vi "Dashboard Main.vi"() -> ()   [LabVIEW 2016]
uses:
  Shared/PID Settings.ctl
  <vilib>/Utility/miscctls.llb/LVRowAndColumnTypeDef.ctl
  <vilib>/event_ctls.llb/eventvkey.ctl
  <vilib>/Rock Robotics/Network Tables/NT Read Numeric Array.vi
  <vilib>/Rock Robotics/WPI/Dashboard/WPI_DashboardLogging Global.vi
panel:
  in  "Camera Settings Right":T1={"Frame Rate"=30, "Compression"=30, "Size"=1, "DB Camera Config"=FALSE} {"Frame Rate" scale=1.0..30.0; "Compression" scale=100.0..-1.0; "Size" items=["640x480", "320x240", "160x120"]}
  in  "Camera Name Right":string(combo)="No Camera Selection"
  out "Camera Info":cluster{"Mbps LED":bool, "Mbps":dbl, "fps":dbl} {"fps" format="%#.1g"; "Mbps" format="%#.1g"}
  in  "Camera Settings":T1={"Frame Rate"=30, "Compression"=30, "Size"=1, "DB Camera Config"=FALSE} {"Frame Rate" scale=1.0..30.0; "Compression" scale=100.0..-1.0; "Size" items=["640x480", "320x240", "160x120"]}
  in  "TCP":refnum<k5>
  in  "Rec Mode":enum32{"Stop", "Record", "Playback"}(radio)
  out "Robot IP":string
  out "Image Message":string="Timeout in Camera Communications"
  in  "Dashboard Tab":T2(tab)
  in  "Select Auto":string(combo)="Select Autonomous ..."
  out "NT Connection":bool
  out "MotorChart R":cluster{"Numeric":dbl, "Numeric":dbl}(graph)
  out "MotorChart L":cluster{"Numeric":dbl, "Numeric":dbl}(graph)
  out "MotorSliders R":cluster{"MotorSlide1":dbl, "MotorSlide2":dbl} {"MotorSlide2" scale=-1.0..1.0 scale format="%#_2e"; "MotorSlide1" scale=-1.0..1.0 scale format="%#_2e"}
  out "MotorSliders L":cluster{"MotorSlide1":dbl, "MotorSlide2":dbl} {"MotorSlide2" scale=-1.0..1.0 scale format="%#_2e"; "MotorSlide1" scale=-1.0..1.0 scale format="%#_2e"}
  out "Gyro":dbl(knob) scale=0.0..360.0
  out "JS1 Z":dbl(slide) scale=-1.0..1.0 scale format="%#_2e"
  out "JS1 Graph":cluster{"X":dbl, "Y":dbl}[](graph)
  out "JS1 Buttons":T3
  out "JS2 Z":dbl(slide) scale=-1.0..1.0 scale format="%#_2e"
  out "JS2 Graph":cluster{"X":dbl, "Y":dbl}[](graph)
  out "JS2 Buttons":T3
  out "Mode":T4(ring)=enum."Auto Disabled"
  out "Camera Image Right":T5(plugin-control)
  in  "DB/String 9":string
  in  "DB/String 8":string
  in  "DB/String 7":string
  in  "DB/String 6":string
  in  "DB/String 5":string
  in  "DB/String 4":string
  in  "DB/String 3":string
  in  "DB/String 2":string
  in  "DB/String 1":string
  in  "DB/String 0":string
  in  "DB/Slider 0":dbl(slide) scale=0.0..5.0
  in  "DB/Slider 1":dbl(slide) scale=0.0..5.0
  in  "DB/Slider 2":dbl(slide) scale=0.0..5.0
  in  "DB/Slider 3":dbl(slide) scale=0.0..5.0
  out "DB/LED 3":bool
  out "DB/LED 2":bool
  out "DB/LED 1":bool
  out "DB/LED 0":bool
  in  "DB/Button 3":bool
  in  "DB/Button 2":bool
  in  "DB/Button 1":bool
  in  "DB/Button 0":bool caption="New Name"
  in  "Custom Tab Control":enum32{"Basic", "Robot Drive"}(tab)
  in  "Save Values":bool
  in  "Drive PID - High":T6
  in  "Left / Right":bool
  out "PID Graph":cluster{"Numeric":dbl, "Numeric":dbl}(graph)
  in  "Drive PID - Low":T6
  in  "Test Slider":dbl(slide) scale=0.0..100.0 scale format="%#_3g"
  in  "On/Off":bool caption="Solenoid"
  in  "Test Name":u16(ring) items=["Select the test to run..."]
  in  "Test Tree":string(tree)
  in  "Motor":cluster{"Value":dbl, "Enable":bool} {"Value" scale=-1.0..1.0 scale format="%#_3g"}
  out "Progress":T7 {"Test Progress" scale=0.0..100.0}
  in  "Rev/Fwd":cluster{"Forward":bool, "Reverse":bool}
  in  "Test Ring":u16(ring) items=["Monochrome", "Color"]
  out "Cmd Status":string
  in  "Execute Command":bool
  in  "Command Params":string[][](table)
  in  "Command Selection":i32(listbox)
  in  "CheckList":i32(listbox)
  out "Tree":string(tree)
  out "Camera Image":T5(plugin-control)
  out "Background":bool
  in  "Camera Name":string(combo)="No Camera Selection"
  # "HW"
  # "HW"
  # "Joysticks"
  # "Drive Motors"
  # "Front"
  # "Right"
  # "Left"
  # "Back"
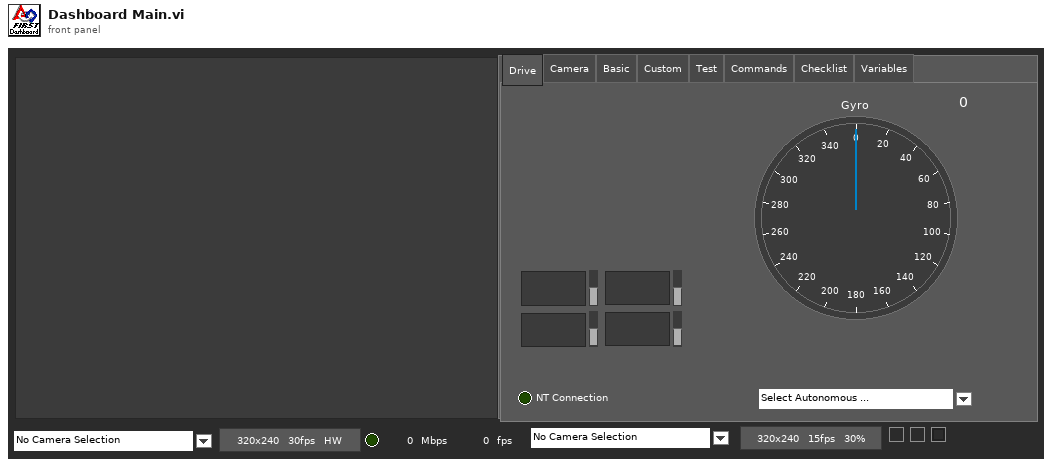
[diagram p1: front panel]
types:
  T1 = cluster{"Frame Rate":i32, "Compression":i32, "Size":u16, "DB Camera Config":bool}
  T2 = enum32{"Drive", "Camera", "Basic", "Custom", "Test", "Commands", "Checklist", "Variables"}
  T3 = cluster{bool, bool, bool, bool, bool, bool, bool, bool, bool, bool, bool, bool}
  T4 = enum8{"Tele-Op Disabled", "Tele-Op Enabled", "Auto Disabled", "Auto Enabled", "Test Disabled", "Test Enabled", "Disconnected", "No Code", "E-Stop"}
  T5 = typedef "IMAQ Image.ctl" = refnum<image>
  T6 = typedef "PID Settings.ctl" = cluster{"D":dbl, "F":dbl, "RR":dbl, "IZ":dbl, "P":dbl, "I":dbl}
  T7 = cluster{"Test Progress":u8, "Test Progress Text":string}
  T8 = typedef "Image Type" = u32
  T9 = cluster{"IDs":cluster{"RPC field ID":u16, "Unique ID":u16}, "String":string}
  T10 = enum32{"Drive", "Basic", "Custom", "Test", "Checklist", "Variables"}
  T11 = cluster{"Error Strings":string, "Disable Counts":cluster{u16, u16}, "Rail Faults":cluster{u16, u16, u16}, "Robot IP":string, "DB Mode":u8, "Event Info":cluster{"Name":string, "Type":u8, "Number":u16, "Replay":u8}}
  T12 = cluster{"Storage":cluster{"Disk Free":u64, "RAM Block":u32, "RAM free":u32}, "CPU Utilization":cluster{"CPU % ISR":sgl, "CPU % Time Crit":sgl, "CPU % Timed Str":sgl, "CPU % High":sgl, "CPU % Above":sgl, "CPU % Normal":sgl, "CPU % Low":sgl}, "CAN":cluster{"% Bus Utilization":sgl, "Bus Off Cnt":u32, "TX_FIFO Full Cnt":u32, "Receive Error Cnt":u8, "Transmit Error Cnt":u8}, "HID":cluster{"HID Outputs":u32, "Rumble Low":u16, "Rumble High":u16}[]}
  T13 = cluster{"Status bits":cluster{"Test Mode":bool, "Autonomous":bool, "Enabled":bool, "Code Start":bool, "Brownout":bool, "Reserved 2":bool, "Reserved 3":bool, "E-Stop":bool}, "Code Trace":cluster{"Disabled":bool, "TeleOp":bool, "Auto":bool, "Test":bool}, "Controller Type":enum16{"unknown", "cRIO", "roboRio"}, "Code?":enum16{"unknown", "noCode", "code"}, "Battery V":dbl}
  T14 = cluster{"Control Bits":cluster{"TestMode":bool, "Autonomous":bool, "Enabled":bool, "FMS Present":bool, bool, bool, bool, "E-Stop":bool}, "Team Station ":u8, "Countdown":sgl, "Joystick Values":cluster{"Axes":dbl[], "Buttons":bool[], "POVs":i16[]}[]}
  T15 = cluster{"Axes":dbl[], "Buttons":bool[], "POVs":i16[]}[]
  T16 = cluster{"Axes":dbl[], "Buttons":bool[], "POVs":i16[]}
  T17 = cluster{"Buttons[0]":bool, "Buttons[1]":bool, "Buttons[2]":bool, "Buttons[3]":bool, "Buttons[4]":bool, "Buttons[5]":bool, "Buttons[6]":bool, "Buttons[7]":bool, "Buttons[8]":bool, "Buttons[9]":bool, "Buttons[10]":bool, "Buttons[11]":bool}
  T18 = cluster{"Camera Image":refnum<vi>, "Dashboard Tab":refnum<vi>, "Background":refnum<vi>, "Rec Mode":refnum<vi>, "Test Slider":refnum<vi>, "On/Off ":refnum<vi>, "Test Ring":refnum<vi>, "Rev/Fwd":refnum<vi>, "Test Name":refnum<vi>, "Motor":refnum<vi>, "Progress":refnum<vi>, "CheckList":refnum<vi>, "Tree":refnum<vi>, "Test Tree":refnum<vi>, "Command Params":refnum<vi>, "Command Selection":refnum<vi>, "Execute Command":refnum<vi>, "Cmd Status":refnum<vi>, "Camera Settings":refnum<vi>, "Camera Name":refnum<vi>, "Camera Info":refnum<vi>, "Camera Settings Right":refnum<vi>, "Camera Name Right":refnum<vi>, "Camera Image Right":refnum<vi>}
  T19 = cluster{"Operation":enum16{"Update", "Clear"}, "Color Box":u32}[]
  T20 = typedef "eventvkey.ctl" = enum16{"ASCII", "Enter", "Return", "Shift", "Ctrl", "Alt", "Cmd", "Opt", "Caps", "NumLock", "Clear", "Break", "Up", "Down", "Left", "Right", "Insert", "Delete", "Home", "End", "PageUp", "PageDown", "Escape", "Help", "Pause", "ScrollLock", "F1", "F2", "F3", "F4", "F5", "F6", "F7", "F8", "F9", "F10", "F11", "F12", "F13", "F14", "F15", "F16", "F17", "F18", "F19", "F20", "F21", "F22", "F23", "F24", "Play", "VolumeUp", "VolumeDown", "Mute", "Two Byte Char"}
  T21 = cluster{"Image Size":bool, "Image Type":bool, "Pixel Value":bool, "ROI Information":bool, "Zoom Factor":bool}
  T22 = cluster{"Operation":enum16{"Update", "Clear"}, "Color Box":u32}
  T23 = typedef "LVRowAndColumnTypeDef.ctl" = cluster{"Row":i32, "Column":i32}
  T24 = cluster{"Shift":bool, "Ctrl":bool, "Alt":bool, "Cmd":bool, "Opt":bool}
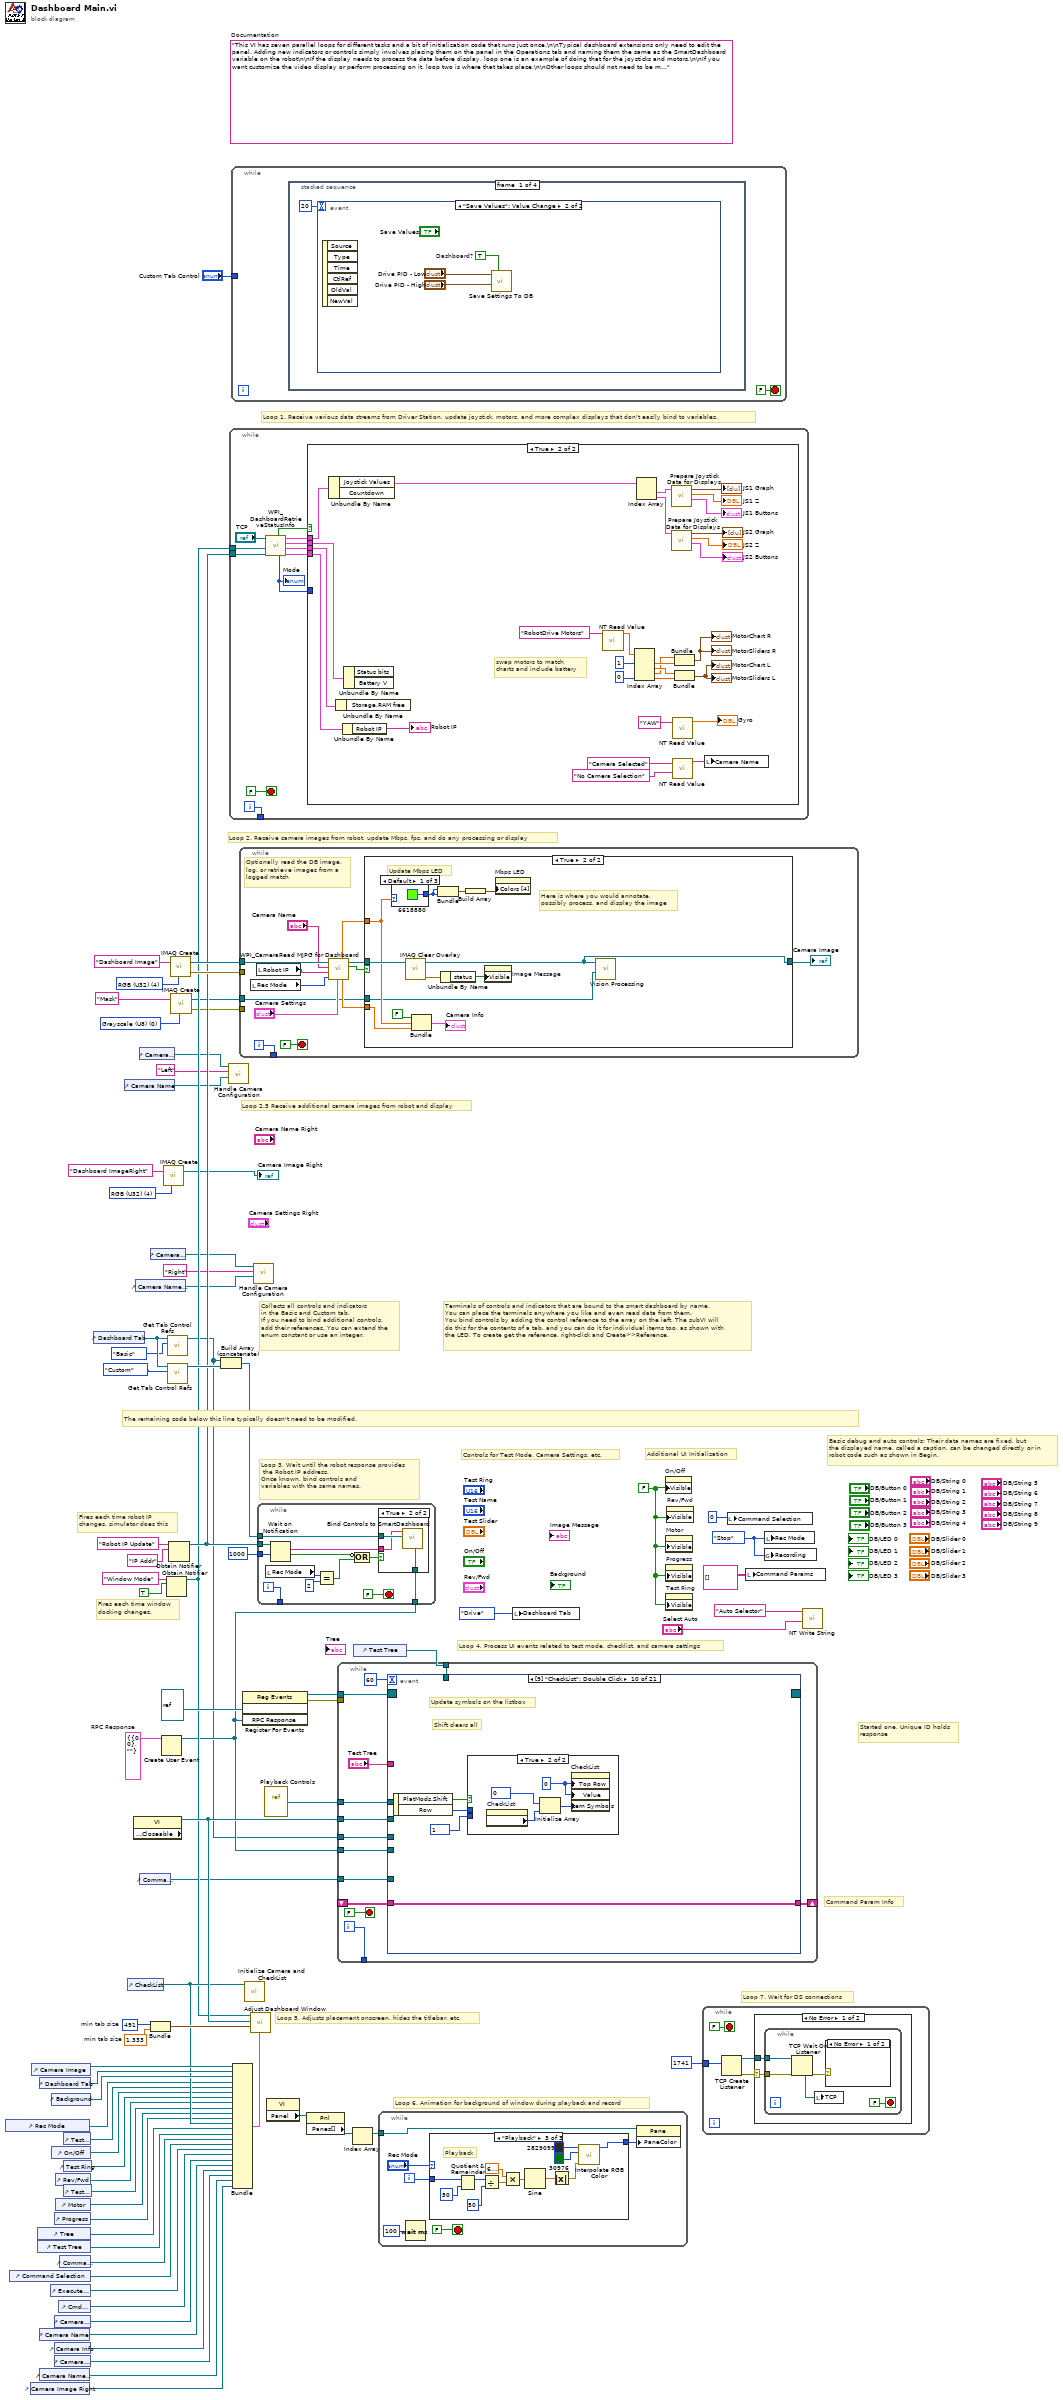
[diagram p0: block diagram]
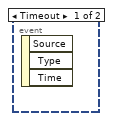
[diagram p2: hidden frame]
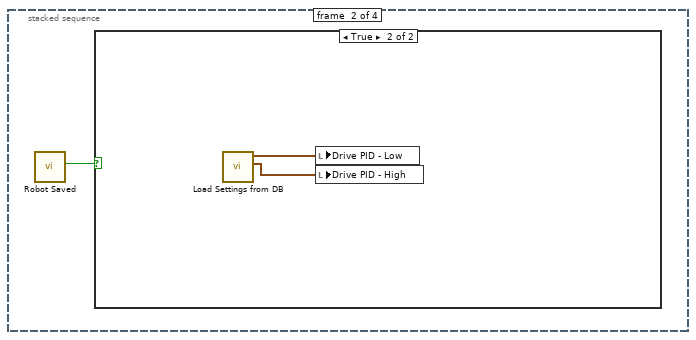
[diagram p3: hidden frame]
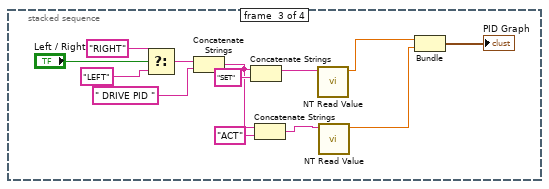
[diagram p5: hidden frame]
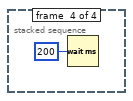
[diagram p6: hidden frame]
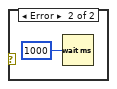
[diagram p7: hidden frame]
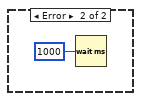
[diagram p8: hidden frame]
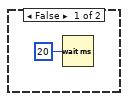
[diagram p9: hidden frame]
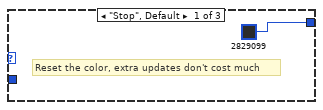
[diagram p10: hidden frame]
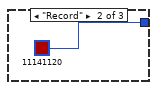
[diagram p11: hidden frame]
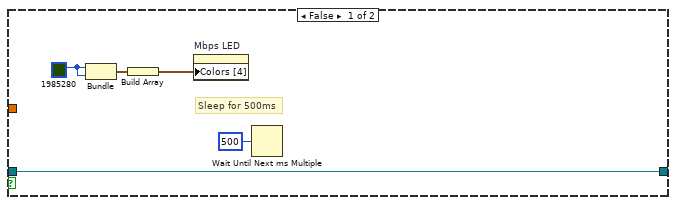
[diagram p13: hidden frame]
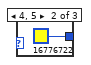
[diagram p14: hidden frame]
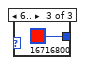
[diagram p15: hidden frame]
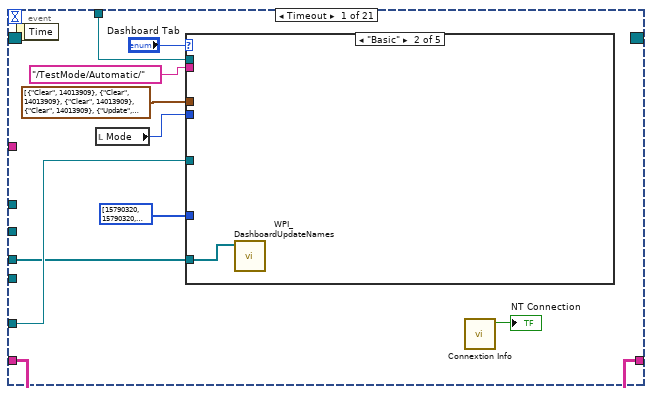
[diagram p16: hidden frame]
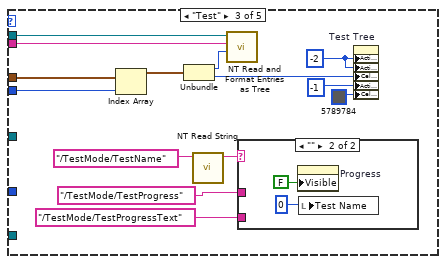
[diagram p18: hidden frame]
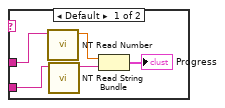
[diagram p19: hidden frame]
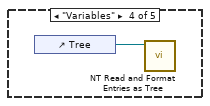
[diagram p20: hidden frame]
diagram:
  w4 = T8 0 items=["Grayscale (U8)", "Grayscale (I16)", "Grayscale (SGL)", "Complex (CSG)", "RGB (U32)", "HSL (U32)", "RGB (U64)", "Grayscale (U16)"] ("Image Type")
  w14 = T8 4 items=["Grayscale (U8)", "Grayscale (I16)", "Grayscale (SGL)", "Complex (CSG)", "RGB (U32)", "HSL (U32)", "RGB (U64)"] ("Image Type")
  w30 = T9 {"IDs"={"RPC field ID"=0, "Unique ID"=0}, "String"=""}  # RPC Response
  w55 = 491  # min tab size
  w54 = 1.333  # min tab size
  w62 = enum32{"Stop", "Record", "Playback"}."Stop" ("Rec Mode")
  w37 = FALSE ("Visible")
  (unwired) "This VI has seven parallel loops for different tasks and a bit of initialization code that runs just once.\n\nTypical dashboard extensions only need to edit the panel. Adding new indicators or controls simply involves placing them on the panel in the Operations tab and naming them the same as the SmartDashboard variable on the robot\n\nIf the display needs to process the data before display, loop one is an example of doing that for the joysticks and motors.\n\nIf you want customize the video display or perform processing on it, loop two is where that takes place.\n\nOther loops should not need to be modified. They are pretty standard, and document the task they perform."  # Documentation
  w79 = T8 4 items=["Grayscale (U8)", "Grayscale (I16)", "Grayscale (SGL)", "Complex (CSG)", "RGB (U32)", "HSL (U32)", "RGB (U64)"] ("Image Type")
  # "Loop 2.5 Receive additional camera images from robot and display"
  # "Command Param Info"
  # "Started one, Unique ID holds\nresponse"
  # "Loop 7. Wait for DS connections"
  # "Basic debug and auto controls: Their data names are fixed, but\nthe displayed name, called a caption, can be changed directly or in\nrobot code such as shown in Begin."
  # "Controls for Test Mode, Camera Settings, etc."
  # "Additional UI Initialization"
  # "Loop 6. Animation for background of window during playback and record"
  # "Fires each time robot IP\nchanges, simulator does this"
  # "Fires each time window\ndocking changes."
  # "Collects all controls and indicators\nin the Basic and Custom tab.\nIf you need to bind additional controls,\nadd their references. You can extend the\nenum constant or use an integer."
  # "The remaining code below this line typically doesn't need to be modified."
  # "Loop 4. Process UI events related to test mode, checklist, and camera settings"
  # "Terminals of controls and indicators that are bound to the smart dashboard by name.\nYou can place the terminals anywhere you like and even read data from them.\nYou bind controls by adding the control reference to the array on the left. The subVI will\ndo this for the contents of a tab, and you can do it for individual items too, as shown with\nthe LED. To create get the reference, right-click and Create>>Reference."
  # "Loop 3. Wait until the robot response provides\n the Robot IP address.\nOnce known, bind controls and\nvariables with the same names."
  # "Loop 5. Adjusts placement onscreen, hides the titlebar, etc."
  # "Loop 1. Receive various data streams from Driver Station, update joystick, motors, and more complex displays that don't easily bind to variables."
  # "Loop 2. Receive camera images from robot, update Mbps, fps, and do any processing or display"
  n1 = control-ref of="Rec Mode"() -> (w43:refnum<vi>)
  n2 = control-ref of="Command Selection"() -> (w29:refnum<vi>)
  n3 = control-ref of="Camera Image Right"() -> (w7:refnum<vi>)
  n4 = control-ref of="Camera Image"() -> (w57:refnum<vi>)
  n5 = control-ref of="Tree"() -> (w47:refnum<vi>)
  n6 = control-ref of="Test Tree"() -> (w46:refnum<vi>)
  n7 = control-ref of="Dashboard Tab"() -> (w56:refnum<vi>)
  n8 = control-ref of="Camera Name"() -> (w20:refnum<vi>)
  n9 = control-ref of="Camera Name Right"() -> (w8:refnum<vi>)
  n10 = control-ref of="Execute Command"() -> (w31:refnum<vi>)
  n11 = control-ref of="Background"() -> (w52:refnum<vi>)
  n12 = control-ref of="On/Off"() -> (w41:refnum<vi>)
  n13 = control-ref of="Progress"() -> (w38:refnum<vi>)
  n14 = control-ref of="Camera Settings"() -> (w21:refnum<vi>)
  n15 = control-ref of="Camera Info"() -> (w19:refnum<vi>)
  n16 = control-ref of="Camera Settings Right"() -> (w9:refnum<vi>)
  n17 = control-ref of="Rev/Fwd"() -> (w39:refnum<vi>)
  n18 = control-ref of="Motor"() -> (w44:refnum<vi>)
  n19 = control-ref of="Cmd Status"() -> (w25:refnum<vi>)
  n20 = control-ref of="Command Params"() -> (w32:refnum<vi>)
  n21 = control-ref of="Test Slider"() -> (w42:refnum<vi>)
  n22 = control-ref of="Test Ring"() -> (w40:refnum<vi>)
  n23 = control-ref of="Test Name"() -> (w45:refnum<vi>)
  n24 = control-ref of="Dashboard Tab"() -> (w60:refnum<vi>)
  n25 = control-ref of="Camera Name"() -> (w22:refnum<vi>)
  n26 = control-ref of="CheckList"() -> (w48:refnum<vi>)
  n27 = property class="VI" props=["Front Panel.Closeable"]() -> (reference out=w61:refnum<vi>)  [unwired: 2 in, 2 out]
  n28 = control-ref of="Camera Name Right"() -> (w12:refnum<vi>)
  n29 = control-ref of="Camera Settings"() -> (w23:refnum<vi>)
  n30 = control-ref of="Command Params"() -> (w24:refnum<vi>)
  n31 = control-ref of="Camera Settings Right"() -> (w13:refnum<vi>)
  n32 = Bundle("min tab size"=w55, "min tab size"=w54) -> (w53:cluster{"min tab size":i32, "min tab size":dbl})  [unwired: 1 in]
  n33 = Create User Event(user event datatype=w30) -> (user event=w26:refnum<user-event>)  [unwired: 1 in, 1 out]
  n34 = call "IMAQ Create"("Image Name"="Dashboard ImageRight", "Image Type"=w14) -> ("New Image"=→"Camera Image Right":T5)  [unwired: 2 in, 2 out]
  n35 = Obtain Notifier(name (unnamed)="Window Mode", notification data type=TRUE) -> (notifier out=w35:refnum<notifier>)  [unwired: 2 in, 2 out]
  n36 = call <vilib>:"Get Tab Control Refs.vi"("Page Index"=T10."Basic" ("Dashboard Tab"), "TabControl in"=w60) -> ("ControlsOnPage"=w18:refnum<vi>[])  [unwired: 9 in]
  n37 = call <vilib>:"Get Tab Control Refs.vi"("Page Index"=T10."Custom" ("Dashboard Tab"), "TabControl in"=w60) -> ("ControlsOnPage"=w59:refnum<vi>[])  [unwired: 9 in]
  n38 = Obtain Notifier(name (unnamed)="Robot IP Update", notification data type="IP Addr" ("name (unnamed)")) -> (notifier out=w36:refnum<notifier>)  [unwired: 2 in, 2 out]
  n39 = call "IMAQ Create"("Image Name"="Dashboard Image", "Image Type"=w79) -> ("New Image"=w77:T5, "error out"=w76:errorcluster)  [unwired: 2 in, 1 out]
  n40 = call "IMAQ Create"("Image Name"="Mask", "Image Type"=w4) -> ("New Image"=w2:T5, "error out"=w1:errorcluster)  [unwired: 2 in, 1 out]
  n41 = Build Array (concatenate)(w18, w59) -> (w58:refnum<vi>[])
  n42 = call "Handle Camera Configuration.vi"("CameraNameRef"=w22, "Camera File Name"="Left", "ClusterRef"=w23) -> ()  [unwired: 9 in]
  n43 = while {
    tunnel: [w89] -> _
    tunnel: w36 -> [w83]
    tunnel: w35 -> [w80]
    i -> [w89]
    stop <- FALSE stop-if-true
    n44 = call <vilib>:"WPI_DashboardRetrieveStatusInfo.vi"("Binding Refnum"=w83, "Window Mode Notifier"=w80, "TCP Cnx"="TCP") -> ("Power and Errors"=w84:T11, "Robot Metrics"=w87:T12, "Status Info"=w88:T13, "Control Info"=w85:T14, "Robot Mode"=w82:T4, "Process?"=w86:bool)  [unwired: 3 in]
    "Mode" <- w82
    n45 = case shown="True" w86 {
      tunnel: w88 -> [_ w120]
      tunnel: w87 -> [_ w119]
      tunnel: w85 -> [_ w118]
      tunnel: w84 -> [_ w117]
      tunnel: w82 -> [_ _]
      frame False {
        n46 = Wait (ms)(milliseconds to wait=u32 20) -> ()  [unwired: 1 out]
      }
      frame True {
        # "swap motors to match\ncharts and include battery"
        n47 = Unbundle By Name(w118) -> ("Joystick Values"=w108:T15)  [unwired: 1 out]
        n48 = Unbundle By Name(w119) -> ()  [unwired: 1 out]
        n49 = Unbundle By Name(w117) -> ("Robot IP"=→"Robot IP":string)
        n50 = Unbundle By Name(w120) -> ()  [unwired: 2 out]
        n51 = call-poly <vilib>:"NT Read Value.vi"("Name"="RobotDrive Motors") -> ("Numeric Array"=w98:dbl[])  [unwired: 9 in, 1 out]
        n52 = Index Array(array=w98, index #1=1, index #4=0) -> (element #1=w112:dbl, element #2=w113:dbl, element #3=w111:dbl, element #4=w116:dbl)  [unwired: 2 in]
        n53 = Index Array(array=w108) -> (element #1=w107:T16, element #2=w103:T16)  [unwired: 2 in]
        n54 = call "Prepare Joystick Data for Displays.vi"("Joystick Values"=w103) -> ("Buttons"=→"JS2 Buttons":T17, "Z Axis"=→"JS2 Z":dbl, "Cartesian Data"=→"JS2 Graph":cluster{"X axis":dbl, "X axis":dbl}[])  [unwired: 8 in]
        n55 = call "Prepare Joystick Data for Displays.vi"("Joystick Values"=w107) -> ("Buttons"=→"JS1 Buttons":T17, "Z Axis"=→"JS1 Z":dbl, "Cartesian Data"=→"JS1 Graph":cluster{"X axis":dbl, "X axis":dbl}[])  [unwired: 8 in]
        n56 = call-poly <vilib>:"NT Read Value.vi"("Name"="YAW") -> ("Numeric"=→"Gyro":dbl)  [unwired: 9 in, 1 out]
        n57 = call-poly <vilib>:"NT Read Value.vi"("Default Value"="No Camera Selection", "Name"="Camera Selected") -> ("String"=w92:string)  [unwired: 8 in, 1 out]
        n58 = Bundle("Numeric"=w111, "Numeric"=w112) -> (→"MotorChart R" →"MotorSliders R":cluster{"Numeric":dbl, "Numeric":dbl})  [unwired: 1 in]
        n59 = Bundle("Numeric"=w113, "Numeric"=w116) -> (→"MotorChart L" →"MotorSliders L":cluster{"Numeric":dbl, "Numeric":dbl})  [unwired: 1 in]
        n60 = local write "Camera Name"(w92) -> ()
      }
    }
  }
  n61 = while {
    tunnel: "Custom Tab Control" -> [_]
    stop <- FALSE stop-if-true
    n62 = stacked-sequence {
      frame #0 {
        n63 = event shown="[1] \"Save Values\": Value Change" {
          selector: _ -> [_ _]
          dyn-events: _ -> [_ _]
          timeout: 20 -> [_ _]
          event Timeout {
            n64 = event-data() -> ()  [unwired: 1 in, 3 out]
          }
          event "Save Values": Value Change {
            w124 = TRUE  # Dashboard?
            n65 = event-data() -> ()  [unwired: 1 in, 6 out]
            n66 = call "Save Settings To DB.vi"("Dashboard?"=w124, "Drive PID - High"="Drive PID - High", "Drive PID - Low"="Drive PID - Low") -> ()  [unwired: 7 in, 2 out]
          }
        }
      }
      frame #1 {
        n67 = call "Robot Saved.vi"() -> ("RB SAVED?"=w126:bool)  [unwired: 10 in, 1 out]
        n68 = case shown="True" w126 {
          frame False {
          }
          frame True {
            n69 = call "Load Settings from DB.vi"() -> ("Drive PID - High (out)"=w127:T6, "Drive PID"=w128:T6)  [unwired: 9 in, 1 out]
            n70 = local write "Drive PID - Low"(w128) -> ()
            n71 = local write "Drive PID - High"(w127) -> ()
          }
        }
      }
      frame #2 {
        n72 = Select(t="RIGHT", s="Left / Right", f="LEFT") -> (s? t:f=w138:string)
        n73 = Concatenate Strings(w138, " DRIVE PID " ("string")) -> (w133:string)
        n74 = Concatenate Strings(w133, "SET" ("string")) -> (w129:string)
        n75 = Concatenate Strings(w133, "ACT" ("string")) -> (w131:string)
        n76 = call-poly <vilib>:"NT Read Value.vi"("Name"=w129) -> ("Numeric"=w136:dbl)  [unwired: 9 in, 1 out]
        n77 = call-poly <vilib>:"NT Read Value.vi"("Name"=w131) -> ("Numeric"=w130:dbl)  [unwired: 9 in, 1 out]
        n78 = Bundle("Numeric"=w136, "Numeric"=w130) -> (→"PID Graph":cluster{"Numeric":dbl, "Numeric":dbl})  [unwired: 1 in]
      }
      frame #3 {
        n79 = Wait (ms)(milliseconds to wait=u32 200) -> ()  [unwired: 1 out]
      }
    }
  }
  n80 = Bundle("Camera Image"=w57, "Dashboard Tab"=w56, "Background"=w52, "Rec Mode"=w43, "Test Slider"=w42, "On/Off"=w41, "Test Ring"=w40, "Rev/Fwd"=w39, "Test Name"=w45, "Motor"=w44, "Progress"=w38, "CheckList"=w48, "Tree"=w47, "Test Tree"=w46, "Command Params"=w32, "Command Selection"=w29, "Execute Command"=w31, "Cmd Status"=w25, "Camera Settings"=w21, "Camera Name"=w20, "Camera Info"=w19, "Camera Settings Right"=w9, "Camera Name Right"=w8, "Camera Image Right"=w7) -> (w49:T18)  [unwired: 1 in]
  n81 = while {
    tunnel: w77 -> [w153]
    tunnel: w76 -> [_]
    tunnel: [w154] -> _
    tunnel: w2 -> [w143]
    tunnel: w1 -> [_]
    i -> [w154]
    stop <- FALSE stop-if-true
    # "Optionally read the DB image,\nlog, or retrieve images from a\nlogged match"
    n82 = local read "Rec Mode"() -> (w149:enum32{"Stop", "Record", "Playback"})
    n83 = local read "Robot IP"() -> (w148:string)
    n84 = call <vilib>:"WPI_CameraRead MJPG for Dashboard.vi"("Camera Settings"="Camera Settings", "Rec Mode"=w149, "Robot IP"=w148, "Camera Name"="Camera Name", "Refnum in"=w153) -> ("Active"=w151:bool, "Refnum out"=w152:T5, "FPS"=w150:dbl, "Bandwidth (Mbps)"=w147:dbl)  [unwired: 3 in]
    n85 = case shown="True" w151 {
      tunnel: w152 -> [w156 w168]
      tunnel: w147 -> [_ w165]
      tunnel: w150 -> [_ w166]
      tunnel: [w156 w161] -> w144
      tunnel: w143 -> [_ w162]
      frame False {
        w158 = u32 1985280 ("Color Box")
        # "Sleep for 500ms"
        n86 = Bundle("Color Box"=w158, "Color Box"=w158) -> (w159:cluster{"Color Box":u32, "Color Box":u32})  [unwired: 1 out]
        n87 = Build Array(w159) -> (w157:cluster{"Color Box":u32, "Color Box":u32}[])
        n88 = property on="Mbps LED" class="Bool (strict)"("Colors [4]"=w157) -> ()  [unwired: 2 in, 2 out]
        n89 = Wait Until Next ms Multiple(millisecond multiple=u32 500) -> ()  [unwired: 1 out]
      }
      frame True {
        # "Here is where you would annotate,\npossibly process, and display the image"
        # "Update Mbps LED"
        n90 = case shown="Default" w165 {
          tunnel: [u32 6618880 ("Color Box") u32 16776722 ("Color Box") u32 16716800 ("Color Box")] -> w169
          frame Default {
          }
          frame 4, 5 {
          }
          frame 6.. {
          }
        }
        n91 = call "IMAQ Clear Overlay"("Image"=w168) -> ("error out"=w171:errorcluster, "Image Out"=w161:T5)  [unwired: 2 in, 7 out]
        n92 = Bundle(FALSE, "Bandwidth (Mbps)"=w165, "FPS"=w166) -> (→"Camera Info":cluster{bool, "Bandwidth (Mbps)":dbl, "FPS":dbl})  [unwired: 1 in]
        n93 = Bundle("Color Box"=w169, "Color Box"=w169) -> (w170:cluster{"Color Box":u32, "Color Box":u32})  [unwired: 1 out]
        n94 = Unbundle By Name(w171) -> ("status"=w172:bool)
        n95 = Build Array(w170) -> (w167:cluster{"Color Box":u32, "Color Box":u32}[])
        n96 = property on="Image Message" class="Str"("Visible"=w172) -> ()  [unwired: 2 in, 2 out]
        n97 = property on="Mbps LED" class="Bool (strict)"("Colors [4]"=w167) -> ()  [unwired: 2 in, 2 out]
        n98 = call "Vision Processing.vi"("Masked Image"=w162, "New Image"=w161) -> ()  [unwired: 10 in]
      }
    }
    "Camera Image" <- w144
  }
  n99 = register-events(refnum<vi> refnum, w26) -> (reference out=w66:refnum<event-registration>, error out=w65:errorcluster)  [unwired: 2 in]
  n100 = call "Initialize Camera and CheckList.vi"("ListBox in"=w48) -> ()  [unwired: 11 in]
  n101 = call "Adjust Dashboard Window.vi"("Sizing Refnums"=w49, "Size Constraints"=w53, "VI"=w61, "WIn Mode"=w35) -> ()  [unwired: 8 in]
  n102 = call "Handle Camera Configuration.vi"("CameraNameRef"=w12, "Camera File Name"="Right", "ClusterRef"=w13) -> ()  [unwired: 9 in]
  n103 = while {
    tunnel: w58 -> [w187]
    tunnel: w36 -> [w185]
    tunnel: [w183] -> _
    tunnel: u32 1000 ("milliseconds to wait") -> [w182]
    tunnel: w26 -> [w176]
    i -> [w183]
    stop <- FALSE stop-if-true
    n104 = local read "Rec Mode"() -> (w178:enum32{"Stop", "Record", "Playback"})
    n105 = Wait on Notification(notifier=w185, timeout in ms (-1)=w182) -> (notification=w184:string, timed out?=w180:bool)  [unwired: 2 in, 2 out]
    n106 = Equal?(x=w178, y=u16 2 ("Rec Mode")) -> (x = y?=w179:bool)
    n107 = Compound Arithmetic op=OR(invert w180, w179) -> (w181:bool)
    n108 = case shown="True" w181 {
      tunnel: w187 -> [_ w190]
      tunnel: w184 -> [_ w189]
      tunnel: w176 -> [_ w188]
      frame False {
      }
      frame True {
        n109 = call <vilib>:"Bind Controls to SmartDashboard.vi"("RPC ref"=w188, "Bound Control Refs"=w190, "Server IP Address"=w189) -> ()  [unwired: 9 in]
      }
    }
  }
  n110 = vi-ref "Playback Controls.vi"() -> (w67:refnum<vi>)
  n111 = property class="VI"() -> ("Panel"=w69:refnum<vi>)  [unwired: 2 in, 2 out]
  n112 = property class="Pnl"(reference=w69) -> ("Panes[]"=w70:refnum<vi>[])  [unwired: 1 in, 2 out]
  n113 = Index Array(array=w70) -> (element=w68:refnum<vi>)  [unwired: 1 in]
  n114 = control-ref of="Test Tree"() -> (w71:refnum<vi>)
  n115 = while {
    tunnel: [w200] -> _
    tunnel: w71 -> [w199]
    tunnel: w67 -> [w198]
    tunnel: w66 -> [w197]
    tunnel: w65 -> [_]
    tunnel: w61 -> [w196]
    tunnel: w26 -> [w195]
    tunnel: w24 -> [w194]
    shift-right: [w193] -> _
    shift-left: _ -> [w192]
    tunnel: w18 -> [w191]
    i -> [w200]
    stop <- FALSE stop-if-true
    n116 = event shown="[9] \"CheckList\": Double Click" {
      selector: w197 -> [_ _ _ _ _ _ _ _ _ _ _ _ _ _ _ _ _ _ _ _ _]
      dyn-events: [_ _ _ _ _ _ _ _ _ _ _ _ _ _ _ _ w456 _ _ _ _] -> _
      timeout: u32 60 ("milliseconds to wait") -> [_ _ _ _ _ _ _ _ _ _ _ _ _ _ _ _ _ _ _ _ _]
      tunnel: w199 -> [w212 _ _ _ _ _ _ _ _ _ _ _ _ _ _ _ _ _ _ _ _]
      tunnel: "Test Tree" -> [_ _ _ _ _ _ _ _ _ _ _ w423 w431 w433 w437 w445 _ _ _ _ _]
      tunnel: w198 -> [_ _ _ _ _ _ _ _ _ _ _ _ _ _ _ _ w458 _ w476 _ _]
      tunnel: w196 -> [_ _ _ _ _ _ _ _ _ _ _ _ _ _ _ _ w454 _ _ _ _]
      tunnel: w195 -> [_ _ _ _ _ _ _ _ _ _ _ _ _ _ _ _ w450 _ _ _ _]
      tunnel: w194 -> [w207 _ _ _ _ _ w374 _ _ _ _ _ _ _ _ _ _ _ _ _ _]
      tunnel: [w206 w251 w353 w358 w367 w371 w372 w381 w391 w398 w410 w422 w429 w432 w436 w444 w449 w471 w473 w477 w488] -> w193
      tunnel: w192 -> [w206 w251 w353 w358 w367 w371 w372 _ _ w398 w410 w422 w429 w432 w436 w444 w449 w471 w473 w477 w488]
      tunnel: w191 -> [w204 _ _ _ _ _ _ _ _ _ _ _ _ _ _ _ _ _ _ _ _]
      event Timeout {
        n117 = event-data() -> ()  [unwired: 1 in, 1 out]
        n118 = local read "Mode"() -> (w209:T4)
        n119 = case shown="\"Basic\"" "Dashboard Tab" {
          tunnel: w212 -> [_ _ w228 _ _]
          tunnel: "/TestMode/Automatic/" ("Name Pattern") -> [_ _ w227 _ _]
          tunnel: T19 [{"Operation"=enum."Clear", "Color Box"=14013909}, {"Operation"=enum."Clear", "Color Box"=14013909}, {"Operation"=enum."Clear", "Color Box"=14013909}, {"Operation"=enum."Clear", "Color Box"=14013909}, {"Operation"=enum."Update", "Color Box"=14013909}, {"Operation"=enum."Update", "Color Box"=16777215}, {"Operation"=enum."Clear", "Color Box"=14013909}, {"Operation"=enum."Clear", "Color Box"=14013909}, {"Operation"=enum."Clear", "Color Box"=14013909}] -> [_ _ w220 _ w244]
          tunnel: w209 -> [_ _ w219 _ w243]
          tunnel: u32[] [15790320, 15790320, 15790320, 15790320, 16777215, 16777215, 15790320, 15790320, 15790320] -> [_ _ _ _ w249]
          tunnel: w207 -> [_ _ _ _ w237]
          tunnel: w204 -> [_ w214 _ _ _]
          frame "Custom", Default {
          }
          frame "Basic" {
            n120 = call <vilib>:"WPI_DashboardUpdateNames.vi"("Controls on Tab"=w214) -> ()  [unwired: 11 in]
          }
          frame "Test" {
            w226 = -2 ("Active Item:Row Number")
            n121 = Index Array(array=w220, index=w219) -> (element=w221:T22)
            n122 = Unbundle(w221) -> ("Operation"=w222:enum16{"Update", "Clear"}, "Color Box"=w223:u32)
            n123 = call <vilib>:"NT Read String.vi"("Name"="/TestMode/TestName") -> ("String"=w217:string)  [unwired: 9 in, 1 out]
            n124 = call <vilib>:"NT Read and Format Entries as Tree.vi"("Operation"=w222, "Name Pattern"=w227, "Tree Refnum"=w228) -> ()  [unwired: 7 in, 2 out]
            n125 = case shown="\"\"" w217 {
              tunnel: "/TestMode/TestProgress" ("Name") -> [w230 _]
              tunnel: "/TestMode/TestProgressText" ("Name") -> [w229 _]
              frame Default {
                n126 = call <vilib>:"NT Read Number.vi"("Name"=w230) -> ("Numeric"=w231:dbl)  [unwired: 9 in, 1 out]
                n127 = call <vilib>:"NT Read String.vi"("Name"=w229) -> ("String"=w232:string)  [unwired: 9 in, 1 out]
                n128 = Bundle("Numeric"=w231, "String"=w232) -> (→"Progress":cluster{"Numeric":dbl, "String":string})  [unwired: 1 in]
              }
              frame "" {
                n129 = property on="Progress" class="Clust (strict)"("Visible"=FALSE) -> ()  [unwired: 2 in, 2 out]
                n130 = local write "Test Name"(u16 0) -> ()
              }
            }
            n131 = property on="Test Tree" class="Tree (strict)"("Active Item Row Number"=w226, "ActiveColNum"=w226, "CellBG"=w223, "Active Item Row Number"=-1 ("Active Item:Row Number"), "CellBG"=u32 5789784 ("Color Box")) -> ()  [unwired: 2 in, 2 out]
          }
          frame "Variables" {
            n132 = control-ref of="Tree"() -> (w236:refnum<vi>)
            n133 = call <vilib>:"NT Read and Format Entries as Tree.vi"("Tree Refnum"=w236) -> ()  [unwired: 9 in, 2 out]
          }
          frame "Commands" {
            w245 = u32 5789784 ("Color Box")
            w246 = T23 {"Row"=-1, "Column"=-2} ("Active Cell:Active Cell")
            w248 = T23 {"Row"=-2, "Column"=-2} ("Active Cell:Active Cell")
            n134 = Index Array(array=w249, index=w243) -> (element=w247:u32)
            n135 = Index Array(array=w244, index=w243) -> (element=w242:T22)
            n136 = Unbundle(w242) -> ("Operation"=w241:enum16{"Update", "Clear"})  [unwired: 1 out]
            n137 = local read "Command Selection"() -> (w240:i32)
            n138 = property on="Command Selection" class="MCListbox (strict)"("ActiveCell"=w248, "CellBG"=w247, "ActiveCell"=w246, "CellBG"=w245) -> ()  [unwired: 2 in, 2 out]
            n139 = call <vilib>:"WPI_DashboardUpdate RPC Info.vi"("Operation"=w241) -> ("update"=w239:bool, "commands"=w238:string[][])  [unwired: 9 in]
            n140 = property on="Command Selection" class="MCListbox (strict)"("ItemNames"=w238) -> ()  [unwired: 2 in, 2 out]
            n141 = property on="Command Params" class="Tbl (strict)"("Active Cell"=w248, "Cell BG Color"=w247, "Active Cell"=w246, "Cell BG Color"=w245) -> ()  [unwired: 2 in, 2 out]
            n142 = call <vilib>:"WPI_DashboardUpdate Command Params.vi"("Update"=w239, "NewVal"=w240, "Commands"=w238, "Param Tbl"=w237) -> ()  [unwired: 7 in, 1 out]
          }
        }
        n143 = call <vilib>:"Connextion Info.vi"() -> ("Connected"=→"NT Connection":bool)  [unwired: 10 in, 1 out]
      }
      event "Test Tree": Value Change {
        # "Show appropriate\ncontrols"
        n144 = event-data() -> ("CtlRef"=w254:refnum<vi>, "NewVal"=w252:string)  [unwired: 1 in]
        n145 = call <vilib>:"WPI_UtilitiesGetTreeIOName.vi"("NewVal"=w252, "TreeControl in"=w254) -> ("I/O Name"=w255:string)  [unwired: 9 in]
        n146 = case shown="\"Camera\"" w255 {
          selector: w255 -> [_ w262 _ w284 w293 _]
          tunnel: w252 -> [_ _ w281 w283 _ w300]
          tunnel: cluster{string[]}[] [{["640x480", "320x240", "160x120"]}, {["Auto", "Fixed indoor", "Fixed outdoor 1", "Fixed outdoor 2", "Fixed fluorescent 1", "Fixed fluorescent 2", "Hold current"]}, {["Auto", "Flicker-free 50 Hz", "Flicker-free 60 Hz", "Hold current"]}, {["None", "Prioritize frame rate", "Prioritize image quality"]}, {["Monochrome", "Color"]}] -> [_ _ _ _ _ w299]
          frame Default {
            w257 = FALSE ("Visible")
            w256 = FALSE ("Visible")
            n147 = property on="Motor" class="Clust (strict)"("Visible"=w256) -> ()  [unwired: 2 in, 2 out]
            n148 = property on="Test Ring" class="Ring (strict)"("Visible"=w256) -> ()  [unwired: 2 in, 2 out]
            n149 = property on="Rev/Fwd" class="Clust (strict)"("Visible"=w257) -> ()  [unwired: 2 in, 2 out]
            n150 = property on="On/Off" class="Bool (strict)"("Visible"=w257) -> ()  [unwired: 2 in, 2 out]
            n151 = property on="Test Slider" class="Slide (strict)"("Visible"=w257) -> ()  [unwired: 2 in, 2 out]
          }
          frame "Analog Out", "Motor", "PWM" {
            w263 = FALSE ("Visible")
            n152 = case shown="\"Analog Out\"" w262 {
              tunnel: [1.0 ("Value") -1.0 ("Value") 0.0 ("Value")] -> w261
              tunnel: [255.0 ("Value") 1.0 ("Value") 5.0 ("Value")] -> w260
              tunnel: [128.0 ("Value") 0.0 ("Value") 0.0 ("Value")] -> w259
              tunnel: [64.0 ("Value") 0.5 ("Value") 1.0 ("Value")] -> w258
              frame "PWM" {
              }
              frame "Motor", Default {
              }
              frame "Analog Out" {
              }
            }
            n153 = property on="Motor" class="Clust (strict)"("Visible"=TRUE) -> ()  [unwired: 2 in, 2 out]
            n154 = property on="Value" class="Slide (strict)"("Value"=w259, "Scale.Minimum"=w261, "Scale.Maximum"=w260, "Scale.Increment"=w258) -> ()  [unwired: 2 in, 2 out]
            n155 = property on="On/Off" class="Bool (strict)"("Visible"=w263) -> ()  [unwired: 2 in, 2 out]
            n156 = property on="Test Slider" class="Slide (strict)"("Visible"=w263) -> ()  [unwired: 2 in, 2 out]
            n157 = property on="Test Ring" class="Ring (strict)"("Visible"=w263) -> ()  [unwired: 2 in, 2 out]
            n158 = property on="Rev/Fwd" class="Clust (strict)"("Visible"=w263) -> ()  [unwired: 2 in, 2 out]
          }
          frame "Servo" {
            w279 = FALSE ("Visible")
            n159 = call <vilib>:"NT Read Number.vi"("Name"=w281) -> ("Numeric"=w280:dbl)  [unwired: 9 in, 1 out]
            n160 = property on="Test Slider" class="Slide (strict)"("Visible"=TRUE, "Scale.Maximum"=170.0 ("Scale.Range:Maximum")) -> ()  [unwired: 2 in, 2 out]
            n161 = local write "Test Slider"(w280) -> ()
            n162 = property on="Motor" class="Clust (strict)"("Visible"=w279) -> ()  [unwired: 2 in, 2 out]
            n163 = property on="Rev/Fwd" class="Clust (strict)"("Visible"=w279) -> ()  [unwired: 2 in, 2 out]
            n164 = property on="On/Off" class="Bool (strict)"("Visible"=w279) -> ()  [unwired: 2 in, 2 out]
            n165 = property on="Test Ring" class="Ring (strict)"("Visible"=w279) -> ()  [unwired: 2 in, 2 out]
          }
          frame "Relay", "Solenoid" {
            w282 = FALSE ("Visible")
            n166 = property on="Motor" class="Clust (strict)"("Visible"=w282) -> ()  [unwired: 2 in, 2 out]
            n167 = property on="Test Slider" class="Slide (strict)"("Visible"=w282) -> ()  [unwired: 2 in, 2 out]
            n168 = Search and Replace String(input string=w283, search string="/Value  **", replace string="/Direction") -> (result string=w289:string)  [unwired: 5 in, 3 out]
            n169 = property on="Test Ring" class="Ring (strict)"("Visible"=w282) -> ()  [unwired: 2 in, 2 out]
            n170 = call <vilib>:"NT Read String.vi"("Name"=w289) -> ("String"=w287:string)  [unwired: 9 in, 1 out]
            n171 = Equal?(x="Both directions", y=w287) -> (x = y?=w285:bool)
            n172 = Not(x=w285) -> (.not. x?=w286:bool)
            n173 = property on="Rev/Fwd" class="Clust (strict)"("Visible"=w285) -> ()  [unwired: 2 in, 2 out]
            n174 = property on="On/Off" class="Bool (strict)"("Visible"=w286, "Caption.Text"=w284) -> ()  [unwired: 2 in, 2 out]
          }
          frame "Compressor", "Digital Out" {
            w292 = FALSE ("Visible")
            # "Get direction and finish"
            n175 = property on="Motor" class="Clust (strict)"("Visible"=w292) -> ()  [unwired: 2 in, 2 out]
            n176 = property on="Test Slider" class="Slide (strict)"("Visible"=w292) -> ()  [unwired: 2 in, 2 out]
            n177 = property on="Test Ring" class="Ring (strict)"("Visible"=w292) -> ()  [unwired: 2 in, 2 out]
            n178 = property on="On/Off" class="Bool (strict)"("Visible"=TRUE, "Caption.Text"=w293) -> ()  [unwired: 2 in, 2 out]
            n179 = property on="Rev/Fwd" class="Clust (strict)"("Visible"=FALSE) -> ()  [unwired: 2 in, 2 out]
          }
          frame "Camera" {
            n180 = call <vilib>:"Get Last Path Segment.vi"("String in"=w300) -> ("String out"=w301:string)  [unwired: 10 in]
            n181 = property on="On/Off" class="Bool (strict)"("Visible"=FALSE) -> ()  [unwired: 2 in, 2 out]
            n182 = property on="Motor" class="Clust (strict)"("Visible"=FALSE) -> ()  [unwired: 2 in, 2 out]
            n183 = property on="Rev/Fwd" class="Clust (strict)"("Visible"=FALSE) -> ()  [unwired: 2 in, 2 out]
            n184 = case shown="\"White Balance  **\"" w301 {
              tunnel: w300 -> [w307 w316 w325 w334 w343 _ w349]
              tunnel: w299 -> [w305 w313 w322 w331 w340 _ _]
              frame "Size  **" {
                n185 = Index Array(array=w305) -> (element=w304:cluster{string[]})  [unwired: 1 in]
                n186 = call <vilib>:"NT Read String.vi"("Name"=w307) -> ("String"=w306:string)  [unwired: 9 in, 1 out]
                n187 = Unbundle(w304) -> (w302:string[])
                n188 = Match First String(2:w302, 3:w306) -> (0:w303:i32)  [unwired: 1 out]
                n189 = property on="Test Ring" class="Ring (strict)"("Value"=w303, "Strings []"=w302) -> ()  [unwired: 2 in, 2 out]
                n190 = property on="Test Ring" class="Ring (strict)"("Visible"=TRUE) -> ()  [unwired: 2 in, 2 out]
                n191 = property on="Test Slider" class="Slide (strict)"("Visible"=FALSE) -> ()  [unwired: 2 in, 2 out]
              }
              frame "White Balance  **" {
                n192 = Index Array(array=w313, index=1) -> (element=w314:cluster{string[]})
                n193 = call <vilib>:"NT Read String.vi"("Name"=w316) -> ("String"=w315:string)  [unwired: 9 in, 1 out]
                n194 = Unbundle(w314) -> (w311:string[])
                n195 = Match First String(2:w311, 3:w315) -> (0:w310:i32)  [unwired: 1 out]
                n196 = property on="Test Ring" class="Ring (strict)"("Value"=w310, "Strings []"=w311) -> ()  [unwired: 2 in, 2 out]
                n197 = property on="Test Ring" class="Ring (strict)"("Visible"=TRUE) -> ()  [unwired: 2 in, 2 out]
                n198 = property on="Test Slider" class="Slide (strict)"("Visible"=FALSE) -> ()  [unwired: 2 in, 2 out]
              }
              frame "Exposure  **" {
                n199 = Index Array(array=w322, index=2) -> (element=w323:cluster{string[]})
                n200 = call <vilib>:"NT Read String.vi"("Name"=w325) -> ("String"=w324:string)  [unwired: 9 in, 1 out]
                n201 = Unbundle(w323) -> (w319:string[])
                n202 = Match First String(2:w319, 3:w324) -> (0:w320:i32)  [unwired: 1 out]
                n203 = property on="Test Ring" class="Ring (strict)"("Value"=w320, "Strings []"=w319) -> ()  [unwired: 2 in, 2 out]
                n204 = property on="Test Ring" class="Ring (strict)"("Visible"=TRUE) -> ()  [unwired: 2 in, 2 out]
                n205 = property on="Test Slider" class="Slide (strict)"("Visible"=FALSE) -> ()  [unwired: 2 in, 2 out]
              }
              frame "Exposure Priority  **" {
                n206 = Index Array(array=w331, index=3) -> (element=w332:cluster{string[]})
                n207 = call <vilib>:"NT Read String.vi"("Name"=w334) -> ("String"=w333:string)  [unwired: 9 in, 1 out]
                n208 = Unbundle(w332) -> (w328:string[])
                n209 = Match First String(2:w328, 3:w333) -> (0:w329:i32)  [unwired: 1 out]
                n210 = property on="Test Ring" class="Ring (strict)"("Value"=w329, "Strings []"=w328) -> ()  [unwired: 2 in, 2 out]
                n211 = property on="Test Ring" class="Ring (strict)"("Visible"=TRUE) -> ()  [unwired: 2 in, 2 out]
                n212 = property on="Test Slider" class="Slide (strict)"("Visible"=FALSE) -> ()  [unwired: 2 in, 2 out]
              }
              frame "Color Enable  **" {
                n213 = Index Array(array=w340, index=4) -> (element=w341:cluster{string[]})
                n214 = call <vilib>:"NT Read String.vi"("Name"=w343) -> ("String"=w342:string)  [unwired: 9 in, 1 out]
                n215 = Unbundle(w341) -> (w337:string[])
                n216 = Match First String(2:w337, 3:w342) -> (0:w338:i32)  [unwired: 1 out]
                n217 = property on="Test Ring" class="Ring (strict)"("Value"=w338, "Strings []"=w337) -> ()  [unwired: 2 in, 2 out]
                n218 = property on="Test Ring" class="Ring (strict)"("Visible"=TRUE) -> ()  [unwired: 2 in, 2 out]
                n219 = property on="Test Slider" class="Slide (strict)"("Visible"=FALSE) -> ()  [unwired: 2 in, 2 out]
              }
              frame Default {
                n220 = property on="Test Ring" class="Ring (strict)"("Visible"=FALSE) -> ()  [unwired: 2 in, 2 out]
                n221 = property on="Test Slider" class="Slide (strict)"("Visible"=FALSE) -> ()  [unwired: 2 in, 2 out]
              }
              frame "Brightness  **", "Color Level  **", "Compression  **", "FPS  **", "Sharpness  **" {
                n222 = call <vilib>:"NT Read Number.vi"("Name"=w349) -> ("Numeric"=w348:dbl)  [unwired: 9 in, 1 out]
                n223 = local write "Test Slider"(w348) -> ()
                n224 = property on="Test Slider" class="Slide (strict)"("Visible"=TRUE, "Scale.Maximum"=100.0 ("Scale.Range:Maximum")) -> ()  [unwired: 2 in, 2 out]
                n225 = property on="Test Ring" class="Ring (strict)"("Visible"=FALSE) -> ()  [unwired: 2 in, 2 out]
              }
            }
          }
        }
        n226 = property on="Progress" class="Clust (strict)"("Visible"=FALSE) -> ()  [unwired: 2 in, 2 out]
      }
      event "Test Name": Mouse Enter {
        # "Populate the ring with the list of tests"
        n227 = event-data() -> ()  [unwired: 1 in, 1 out]
        n228 = call <vilib>:"NT Read String Array.vi"("Name"="/TestMode/TestList") -> ("String Array"=w357:string[])  [unwired: 9 in, 1 out]
        n229 = Build Array (concatenate)("Select the test to run...", w357) -> (w356:string[])
        n230 = property on="Test Name" class="Ring (strict)"("Strings []"=w356) -> ()  [unwired: 2 in, 2 out]
      }
      event "Test Name": Value Change {
        w359 = FALSE ("Visible")
        # "Tell the robot the test name to run"
        n231 = event-data() -> ("NewVal"=w363:u16)  [unwired: 1 in]
        n232 = property on="Test Name" class="Ring (strict)"() -> ("Strings []"=w364:string[])  [unwired: 2 in, 2 out]
        n233 = local write "Progress"(T7 {"Test Progress"=0, "Test Progress Text"=""} ("Progress")) -> ()
        n234 = Index Array(array=w364, index=w363) -> (element=w362:string)
        n235 = call <vilib>:"NT Write String.vi"("String"=w362, "Name"="/TestMode/TestName") -> ()  [unwired: 9 in, 1 out]
        n236 = property on="Progress" class="Clust (strict)"("Visible"=TRUE) -> ()  [unwired: 2 in, 2 out]
        n237 = property on="Motor" class="Clust (strict)"("Visible"=w359) -> ()  [unwired: 2 in, 2 out]
        n238 = property on="Test Slider" class="Slide (strict)"("Visible"=w359) -> ()  [unwired: 2 in, 2 out]
        n239 = property on="On/Off" class="Bool (strict)"("Visible"=w359) -> ()  [unwired: 2 in, 2 out]
        n240 = property on="Rev/Fwd" class="Clust (strict)"("Visible"=w359) -> ()  [unwired: 2 in, 2 out]
        n241 = property on="Test Ring" class="Ring (strict)"("Visible"=w359) -> ()  [unwired: 2 in, 2 out]
      }
      event "Select Auto": Mouse Enter {
        # "Populate the combo box with the list of autonomous options"
        n242 = event-data() -> ()  [unwired: 1 in, 1 out]
        n243 = call <vilib>:"NT Read String Array.vi"("Name"="Auto List") -> ("String Array"=w366:string[])  [unwired: 9 in, 1 out]
        n244 = property on="Select Auto" class="CmbBox"("Strings[]"=w366) -> ()  [unwired: 2 in, 2 out]
      }
      event "Select Auto": Value Change {
        # "User modified the Auto Selection. Write to NT variable so robot knows."
        n245 = event-data() -> ("NewVal"=w369:string)  [unwired: 1 in]
        n246 = call <vilib>:"NT Write String.vi"("String"=w369, "Name"="Auto Selector") -> ()  [unwired: 9 in, 1 out]
      }
      event "Command Selection": Value Change {
        # "Get the params and show in table"
        n247 = event-data() -> ("NewVal"=w375:i32)  [unwired: 1 in]
        n248 = property on="Command Selection" class="MCListbox (strict)"() -> ("ItemNames"=w373:string[][])  [unwired: 2 in, 2 out]
        n249 = call <vilib>:"WPI_DashboardUpdate Command Params.vi"("NewVal"=w375, "Commands"=w373, "Param Tbl"=w374) -> ()  [unwired: 8 in, 1 out]
      }
      event "Execute Command": Value Change {
        # "Started one, Unique ID holds\nresponse"
        n250 = event-data() -> ()  [unwired: 1 in, 1 out]
        n251 = property on="Command Selection" class="MCListbox (strict)"() -> ("ItemNames"=w386:string[][])  [unwired: 2 in, 2 out]
        n252 = Index Array(array=w386, index (row)="Command Selection", index (col)=0) -> (element=w384:string)
        n253 = call <vilib>:"Invoke Commands.vi"("Command Params"="Command Params", "Function Name"=w384) -> ("Params"=w380:u8, "Started"=w379:bool)  [unwired: 7 in, 1 out]
        n254 = Array Subset(array="Command Params", length (row)=w380) -> (w381:string[][])  [unwired: 3 in]
        n255 = Select(t="Executing" ("Cmd Status"), s=w379, f="" ("Cmd Status")) -> (s? t:f=→"Cmd Status":string)
      }
      event "Command Selection": Double Click {
        n256 = event-data() -> ("Row"=w394:i32)  [unwired: 1 in]
        n257 = property on="Command Selection" class="MCListbox (strict)"() -> ("ItemNames"=w397:string[][])  [unwired: 2 in, 2 out]
        n258 = local read "Command Params"() -> (w393:string[][])
        n259 = Index Array(array=w397, index (row)=w394, index (col)=0) -> (element=w395:string)
        n260 = call <vilib>:"Invoke Commands.vi"("Command Params"=w393, "Function Name"=w395) -> ("Params"=w392:u8, "Started"=w387:bool)  [unwired: 7 in, 1 out]
        n261 = Array Subset(array=w393, length (row)=w392) -> (w391:string[][])  [unwired: 3 in]
        n262 = Select(t="Executing" ("Cmd Status"), s=w387, f="" ("Cmd Status")) -> (s? t:f=w388:string)
        n263 = local write "Cmd Status"(w388) -> ()
      }
      event "CheckList": Double Click {
        # "Shift clears all"
        # "Update symbols on the listbox"
        n264 = event-data() -> ("PlatMods.Shift"=w399:bool, "Row"=w401:i32)  [unwired: 1 in]
        n265 = case shown="True" w399 {
          tunnel: w401 -> [w405 _]
          tunnel: 1 -> [w404 _]
          frame False {
            n266 = property on="CheckList" class="LstBox (strict)"() -> ("Item Symbols"=w403:i32[])  [unwired: 2 in, 2 out]
            n267 = Replace Array Subset(array=w403, new element=w404, index=w405) -> (w402:i32[])
            n268 = property on="CheckList" class="LstBox (strict)"("Item Symbols"=w402) -> ()  [unwired: 2 in, 2 out]
          }
          frame True {
            w406 = 0 ("Top Row")
            n269 = property on="CheckList" class="LstBox (strict)"() -> ("Number of Rows"=w408:u32)  [unwired: 2 in, 2 out]
            n270 = Initialize Array(0, w408) -> (w407:i32[])
            n271 = property on="CheckList" class="LstBox (strict)"("Top Row"=w406, "Value"=w406, "Item Symbols"=w407) -> ()  [unwired: 2 in, 2 out]
          }
        }
      }
      event "CheckList": Key Down {
        # "Update symbols on the listbox\nLeft and right keys check and uncheck"
        n272 = event-data() -> ("VKey"=w412:T20)  [unwired: 1 in]
        n273 = case shown="\"Left\", \"Right\"" w412 {
          selector: w412 -> [w417 _]
          tunnel: eventvkey."Left" ("VKey") -> [w415 _]
          frame "Left", "Right" {
            n274 = Equal?(x=w415, y=w417) -> (x = y?=w416:bool)
            n275 = Select(t=0, s=w416, f=1) -> (s? t:f=w418:i32)
            n276 = property on="CheckList" class="LstBox (strict)"() -> ("Item Symbols"=w421:i32[])  [unwired: 2 in, 2 out]
            n277 = Replace Array Subset(array=w421, new element=w418, index="CheckList") -> (w420:i32[])
            n278 = property on="CheckList" class="LstBox (strict)"("Item Symbols"=w420) -> ()  [unwired: 2 in, 2 out]
          }
          frame Default {
          }
        }
      }
      event "Motor.Enable": Value Change {
        # "When the test mode otor enable helper is set, update that\ntree row item's value"
        n279 = event-data() -> ("NewVal"=w427:bool)  [unwired: 1 in]
        n280 = Unbundle("Motor") -> ("Value"=w426:dbl)  [unwired: 1 out]
        n281 = Select(t=w426, s=w427, f=0.0) -> (s? t:f=w424:dbl)
        n282 = call <vilib>:"NT Write Number.vi"("Numeric"=w424, "Name"=w423) -> ()  [unwired: 9 in, 1 out]
      }
      event "Test Slider": Value Change {
        # "When the test mode slider helper is set, update that\ntree row item's value"
        n283 = event-data() -> ("NewVal"=w430:dbl)  [unwired: 1 in]
        n284 = call <vilib>:"NT Write Number.vi"("Numeric"=w430, "Name"=w431) -> ()  [unwired: 9 in, 1 out]
      }
      event "On/Off": Value Change {
        # "When the test mode on/off helper value is set, update that\ntree row item's value"
        n285 = event-data() -> ("NewVal"=w435:bool)  [unwired: 1 in]
        n286 = Boolean To (0,1)(Boolean=w435) -> (0, 1=w434:i16)
        n287 = call <vilib>:"NT Write Number.vi"("Numeric"=w434, "Name"=w433) -> ()  [unwired: 9 in, 1 out]
      }
      event "Rev/Fwd": Value Change {
        # "When the test mode helper value for relays is set, update that\ntree row item's value"
        n288 = event-data() -> ("NewVal.Forward"=w443:bool, "NewVal.Reverse"=w442:bool)  [unwired: 1 in]
        n289 = Boolean To (0,1)(Boolean=w443) -> (0, 1=w439:i16)
        n290 = Boolean To (0,1)(Boolean=w442) -> (0, 1=w441:i16)
        n291 = Negate(x=w441) -> (-x=w440:i16)
        n292 = Add(x=w439, y=w440) -> (x+y=w438:i16)
        n293 = call <vilib>:"NT Write Number.vi"("Numeric"=w438, "Name"=w437) -> ()  [unwired: 9 in, 1 out]
      }
      event "Test Ring": Value Change {
        # "When a test mode helper value is selected from the ring,\nset the tree item's variable to the string value"
        n294 = event-data() -> ("NewVal"=w447:u16)  [unwired: 1 in]
        n295 = property on="Test Ring" class="Ring (strict)"() -> ("Strings []"=w448:string[])  [unwired: 2 in, 2 out]
        n296 = Index Array(array=w448, index=w447) -> (element=w446:string)
        n297 = call <vilib>:"NT Write String.vi"("String"=w446, "Name"=w445) -> ()  [unwired: 9 in, 1 out]
      }
      event "Rec Mode": Value Change {
        # "Update globals for recording mode and path to read log from.\nClear when logging and let NetworkTables set path for vision to\nuse."
        n298 = event-data() -> ("NewVal"=w459:enum32{"Stop", "Record", "Playback"})  [unwired: 1 in]
        n299 = global write "WPI_DashboardLogging Global.vi" "Logging Filename"(path "") -> ()
        n300 = global write "WPI_DashboardLogging Global.vi" "Recording"(w459) -> ()
        n301 = case shown="\"Playback\"" w459 {
          tunnel: w458 -> [_ w461 w470]
          tunnel: [_ _ w469] -> w456
          tunnel: [_ _ w468] -> _
          tunnel: w454 -> [_ _ w466]
          tunnel: cluster{i32, i32} {-250, 170} -> [_ _ w465]
          tunnel: [_ _ T21 {"Image Size"=TRUE, "Image Type"=TRUE, "Pixel Value"=TRUE, "ROI Information"=TRUE, "Zoom Factor"=FALSE} ("Image Information Shown:All Elements")] -> w452
          tunnel: [_ _ TRUE ("Zoom Factor")] -> w451
          tunnel: w450 -> [_ _ w462]
          frame Default {
          }
          frame "Stop", "Record" {
            # "Place Window too"
            n302 = invoke class="VI" method="FP.Close"(reference=w461) -> (reference out=w460:refnum<vi>)  [unwired: 2 in, 2 out]
            n303 = invoke class="VI" method="Abort VI"(reference=w460) -> ()  [unwired: 2 in, 3 out]
          }
          frame "Playback" {
            n304 = call "Open Playback Panel.vi"("Offset"=w465, "DB VI Ref"=w466, "Playback in"=w470) -> ("Playback out"=w467:refnum<vi>)  [unwired: 8 in]
            n305 = register-events(w467, w462) -> (reference out=w469:refnum<event-registration>, error out=w468:errorcluster)  [unwired: 2 in]
          }
        }
        n306 = property on="Camera Image" class="ImageControl"("Image Information Shown"=w452, "Image Information Visible"=w451) -> ()  [unwired: 2 in, 2 out]
        n307 = call <vilib>:"WPI_DashboardNT Log FieldName Cache.vi"("Operation"=enum16{"Lookup/Add", "Index", "Clear"}."Clear") -> ()  [unwired: 8 in, 3 out]
      }
      event Panel Close {
        w472 = enum32{"Stop", "Record", "Playback"}."Stop" ("Rec Mode")
        # "Playback window has been closed, abort"
        n308 = event-data() -> ()  [unwired: 1 in, 4 out]
        n309 = local write "Rec Mode"(w472) -> ()
        n310 = global write "WPI_DashboardLogging Global.vi" "Recording"(w472) -> ()
      }
      event Panel Close {
        # "Abort playback window and ourself"
        n311 = event-data() -> ()  [unwired: 1 in, 4 out]
        n312 = invoke class="VI" method="FP.Close"(reference=w476) -> (reference out=w475:refnum<vi>)  [unwired: 2 in, 2 out]
        n313 = invoke class="VI" method="Abort VI"(reference=w475) -> (error out=w474:errorcluster)  [unwired: 2 in, 2 out]
        n314 = invoke class="VI" method="Abort VI"(error in=w474) -> ()  [unwired: 2 in, 3 out]
      }
      event User Event {
        n315 = event-data() -> ("IDs"=w483:cluster{"RPC field ID":u16, "Unique ID":u16}, "String"=w482:string)  [unwired: 1 in]
        n316 = Bundle("IDs"=w483, "String"=w482) -> (w481:T9)  [unwired: 1 in]
        n317 = call <vilib>:"Retrieve RPC Response.vi"("RPC Response"=w481) -> ("Output"=w479:string[][])  [unwired: 10 in]
        n318 = Build Array (concatenate)(w477, w479) -> (w478:string[][])
        n319 = local write "Command Params"(w478) -> ()
        n320 = local write "Cmd Status"("" ("Cmd Status")) -> ()
      }
      event "Tree": Double Click {
        n321 = event-data() -> ("PlatMods"=w487:T24, "Tag"=w486:string)  [unwired: 1 in]
        n322 = Unbundle(w487) -> ("Shift"=w485:bool)  [unwired: 4 out]
        n323 = Not(x=w485) -> (.not. x?=w484:bool)
        n324 = call <vilib>:"NT Update Persistence.vi"("Persistence"=w484, "Name"=w486) -> ()  [unwired: 9 in, 1 out]
      }
    }
  }
  n325 = while {
    tunnel: w68 -> [w490]
    i -> [w493]
    stop <- FALSE stop-if-true
    n326 = Wait (ms)(milliseconds to wait=u32 100) -> ()  [unwired: 1 out]
    n327 = case shown="\"Playback\"" "Rec Mode" {
      tunnel: w493 -> [_ _ w508]
      tunnel: [u32 2829099 ("Base Color") u32 11141120 ("Target Color") w497] -> w489
      frame "Stop", Default {
        # "Reset the color, extra updates don't cost much"
      }
      frame "Record" {
      }
      frame "Playback" {
        # "Playback"
        n328 = Quotient & Remainder(x=w508, y=u32 50 ("milliseconds to wait")) -> (x-y*floor(x/y)=w504:u32)  [unwired: 1 out]
        n329 = Divide(x=w504, y=u32 50 ("milliseconds to wait")) -> (x/y=w501:dbl)
        n330 = Multiply(x=6.283185307179586, y=w501) -> (x*y=w506:dbl)
        n331 = Sine(x=w506) -> (sin(x)=w505:dbl)
        n332 = Absolute Value(x=w505) -> (abs(x)=w498:dbl)
        n333 = call "Interpolate RGB Color.vi"("Proportion"=w498, "Target Color"=u32 30976, "Base Color"=u32 2829099) -> ("Result Color"=w497:u32)  [unwired: 8 in]
      }
    }
    n334 = property class="Pane"(reference=w490, "PaneColor"=w489) -> ()  [unwired: 1 in, 2 out]
  }
  n335 = local write "Dashboard Tab"(T2."Drive" ("Dashboard Tab")) -> ()
  n336 = property on="On/Off" class="Bool (strict)"("Visible"=w37) -> ()  [unwired: 2 in, 2 out]
  n337 = property on="Motor" class="Clust (strict)"("Visible"=w37) -> ()  [unwired: 2 in, 2 out]
  n338 = property on="Progress" class="Clust (strict)"("Visible"=w37) -> ()  [unwired: 2 in, 2 out]
  n339 = property on="Test Ring" class="Ring (strict)"("Visible"=w37) -> ()  [unwired: 2 in, 2 out]
  n340 = property on="Rev/Fwd" class="Clust (strict)"("Visible"=w37) -> ()  [unwired: 2 in, 2 out]
  n341 = while {
    tunnel: u16 1741 ("timeout ms (25000)") -> [w510]
    stop <- FALSE stop-if-true
    n342 = TCP Create Listener(10:w510) -> (0:w509:errorcluster, 3:w511:refnum<k5>)  [unwired: 4 in, 1 out]
    n343 = case shown="No Error" w509 {
      selector: w509 -> [w513 _]
      tunnel: w511 -> [w514 _]
      frame No Error {
        n344 = while {
          tunnel: w514 -> [w517]
          tunnel: w513 -> [w516]
          stop <- FALSE stop-if-true
          n345 = TCP Wait On Listener(8:w516, 11:w517) -> (0:w518:errorcluster, 4:w519:refnum<k5>)  [unwired: 2 in, 3 out]
          n346 = local write "TCP"(w519) -> ()
          n347 = case shown="No Error" w518 {
            frame No Error {
            }
            frame Error {
              n348 = Wait (ms)(milliseconds to wait=u32 1000) -> ()  [unwired: 1 out]
            }
          }
        }
      }
      frame Error {
        n349 = Wait (ms)(milliseconds to wait=u32 1000) -> ()  [unwired: 1 out]
      }
    }
  }
  n350 = local write "Command Selection"(u16 0 ("milliseconds to wait")) -> ()
  n351 = local write "Command Params"(string[][] [] ("Command Params")) -> ()
  n352 = global write "WPI_DashboardLogging Global.vi" "Recording"(w62) -> ()
  n353 = local write "Rec Mode"(w62) -> ()
  n354 = call <vilib>:"NT Write String.vi"("String"="Select Auto", "Name"="Auto Selector") -> ()  [unwired: 9 in, 1 out]
